vi "初机号 1.vi"() -> ()   [LabVIEW 2022 SP3]
uses:
  <vilib>/DAQmx/write.llb/DAQmx Write (Digital Bool 1Line 1Point).vi
  <vilib>/DAQmx/read.llb/DAQmx Read (Analog Wfm 1Chan NSamp).vi
  <vilib>/DAQmx/create/channels.llb/DAQmx Create Channel (AI-Voltage-Basic).vi
  <vilib>/DAQmx/configure/timing.llb/DAQmx Timing (Sample Clock).vi
  <vilib>/DAQmx/create/channels.llb/DAQmx Create Channel (DO-Digital Output).vi
  <vilib>/DAQmx/miscellaneous.llb/DAQmx Fill In Error Info.vi
panel:
  out "充电指示灯":bool
  out "运行指示灯":bool
  in  "文件名":string
  in  "directory":path caption="目录"
  out "输出波形":waveform(dbl)(graph)
  in  "?":bool
  in  "充电":bool
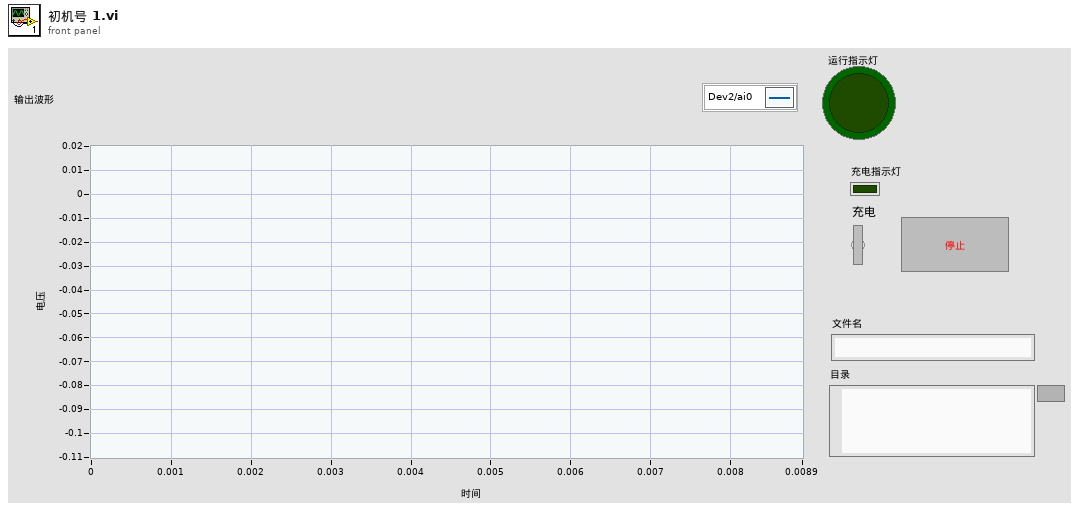
[diagram p1: front panel]
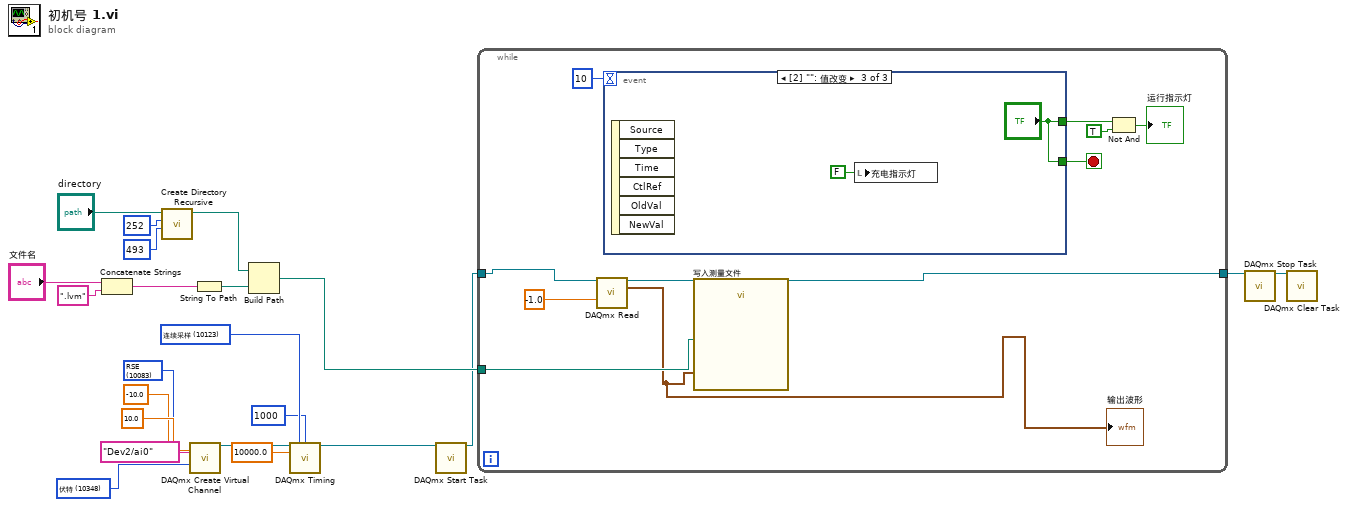
[diagram p0: block diagram]
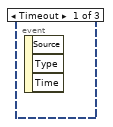
[diagram p2: hidden frame]
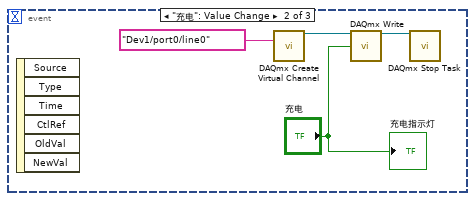
[diagram p3: hidden frame]
diagram:
  w5 = 10123 items=["有限采样"=10178, "连续采样"=10123, "硬件定时单点"=12522] ("sample mode")
  w19 = 10083 items=["默认"=-1, "RSE"=10083, "NRSE"=10078, "差分"=10106, "伪差分"=12529] ("input terminal configuration")
  w22 = 10348 items=["伏特"=10348, "来自自定义换算"=10065] ("units")
  n1 = Concatenate Strings("文件名", ".lvm" ("字符串")) -> (w10:string)
  n2 = call <vilib>:"Create Directory Recursive.vi"("permissions"=i16 493, "maximum path length"=252, "directory"="directory") -> ("directory copy"=w8:path)  [unwired: 2 in, 2 out]
  n3 = call-poly <vilib>:"DAQmx Create Virtual Channel.vi"("maximum value"=10.0, "minimum value"=-10.0, "input terminal configuration"=w19, "physical channels"=tag "Dev2/ai0", "units"=w22) -> ("task out"=w6:refnum<k21>)  [unwired: 9 in, 1 out]
  n4 = String To Path(string=w10) -> (path=w13:path)
  n5 = Build Path(base path=w8, name or relative path=w13) -> (appended path=w9:path)
  n6 = call-poly <vilib>:"DAQmx Timing.vi"("task/channels in"=w6, "sample mode"=w5, "samples per channel"=1000, "rate"=10000.0) -> ("task out"=w1:refnum<k21>)  [unwired: 10 in, 1 out]
  n7 = call <vilib>:"DAQmx Start Task.vi"("task/channels in"=w1) -> ("task out"=w7:refnum<k21>)  [unwired: 13 in, 1 out]
  n8 = while {
    tunnel: w7 -> [w24]
    tunnel: [w29] -> w18
    tunnel: w9 -> [w28]
    stop <- w32 stop-if-true
    n9 = call-poly <vilib>:"DAQmx Read.vi"("task/channels in"=w24, "timeout"=-1.0) -> ("task out"=w29:refnum<k21>, "data"=w23:waveform(dbl))  [unwired: 11 in, 1 out]
    "输出波形" <- w23
    n10 = event shown="[2] \"\": 值改变" {
      selector: _ -> [_ _ _]
      dyn-events: _ -> [_ _ _]
      timeout: 10 -> [_ _ _]
      tunnel: [_ _ "?"] -> w32
      tunnel: [_ _ "?"] -> w27
      event Timeout {
        n11 = event-data() -> ()  [unwired: 1 in, 3 out]
      }
      event "充电": Value Change {
        n12 = event-data() -> ()  [unwired: 1 in, 6 out]
        n13 = call-poly <vilib>:"DAQmx Create Virtual Channel.vi"("lines"=tag "Dev1/port0/line0") -> ("task out"=w36:refnum<k21>)  [unwired: 13 in, 1 out]
        n14 = call-poly <vilib>:"DAQmx Write.vi"("task/channels in"=w36, "data"="充电") -> ("task out"=w34:refnum<k21>)  [unwired: 11 in, 2 out]
        n15 = call <vilib>:"DAQmx Stop Task.vi"("task/channels in"=w34) -> ()  [unwired: 13 in, 2 out]
        "充电指示灯" <- "充电"
      }
      event Value Change {
        n16 = event-data() -> ()  [unwired: 1 in, 6 out]
        n17 = local write "充电指示灯"(FALSE ("充电指示灯")) -> ()
      }
    }
    n18 = call "写入测量文件"("Signals"=w23, "Filename"=w28) -> ()  [unwired: 15 in, 3 out]
    n19 = Not And(1:TRUE ("y"), 2:w27) -> (0:→"运行指示灯":bool)
  }
  n20 = call <vilib>:"DAQmx Stop Task.vi"("task/channels in"=w18) -> ("task out"=w17:refnum<k21>)  [unwired: 13 in, 1 out]
  n21 = call <vilib>:"DAQmx Clear Task.vi"("task in"=w17) -> ()  [unwired: 14 in, 1 out]
